vi "Read Level.vi"(8 "error in (no error)":errorcluster, 11 "SpecAnBase in":refnum<class "SpecAnBase.lvclass">) -> (0 "error out":errorcluster, 2 "Level":T1, 3 "SpecAnBase out":refnum<class "SpecAnBase.lvclass">)   [LabVIEW 2014, in "SpecAnPlugins.lvlib" / "SpecAnBase.lvclass"]
uses:
  SpecAnBase.lvclass
  SpecAnBase.lvclass/SpecAnBase.ctl
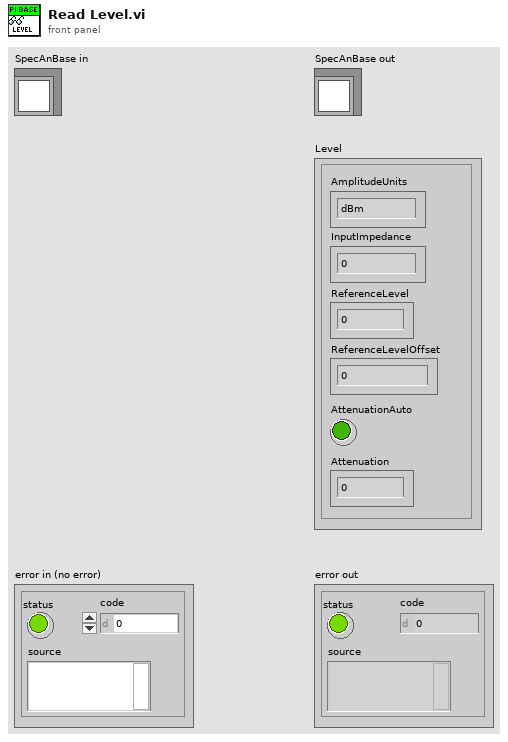
[diagram p1: front panel]
types:
  T1 = cluster{"InputImpedance":dbl, "AttenuationAuto":bool, "AmplitudeUnits":enum16{"dBm", "dBmV", "dBuV", "Volt", "Watt"}, "ReferenceLevel":dbl, "Attenuation":dbl, "ReferenceLevelOffset":dbl}
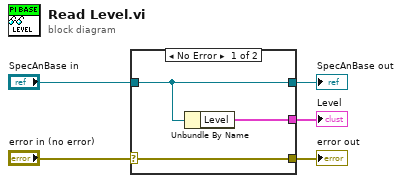
[diagram p0: block diagram]
diagram:
  n1 = case shown="No Error" "error in (no error)" {
    selector: "error in (no error)" -> [w8 w9]
    tunnel: [w8 w9] -> w4
    tunnel: [w7 w10] -> w2
    tunnel: "SpecAnBase in" -> [w7 w10]
    tunnel: [w6 _] -> w1
    frame No Error {
      n2 = Unbundle By Name(w7) -> ("Level"=w6:T1)
    }
    frame Error {
    }
  }
  "error out" <- w4
  "SpecAnBase out" <- w2
  "Level" <- w1
